vi "d7seg.vi"(0 "Numeric":u8 max=9 step=1) -> (19 "appended array":bool[](array[boolean]), 20 "a":bool, 21 "b":bool, 22 "c":bool, 23 "d":bool, 24 "e":bool, 25 "f":bool, 26 "g":bool, 27 "h":bool)   [LabVIEW 2023]
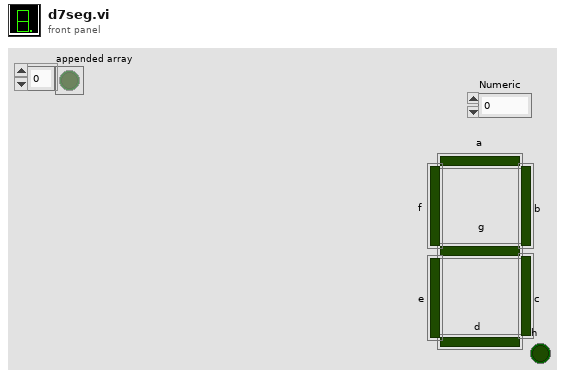
[diagram p1: front panel]
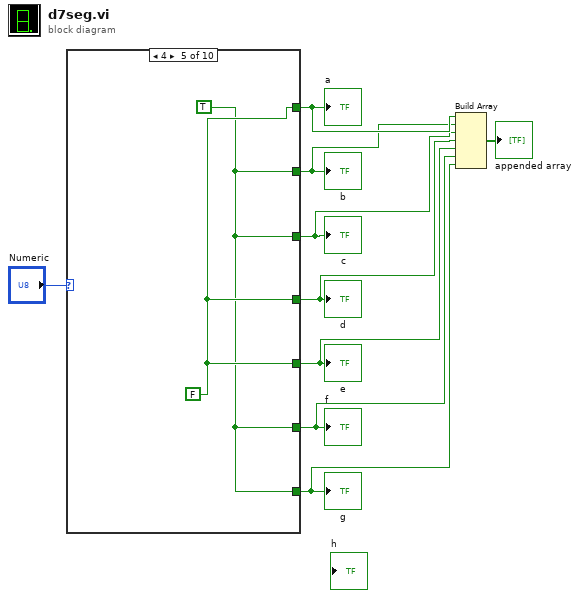
[diagram p0: block diagram]
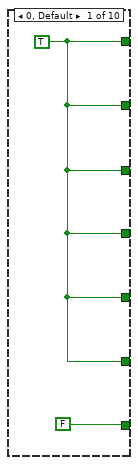
[diagram p2: hidden frame]
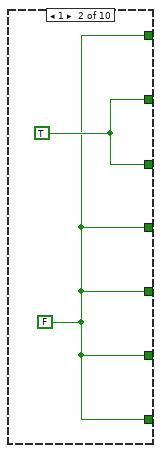
[diagram p3: hidden frame]
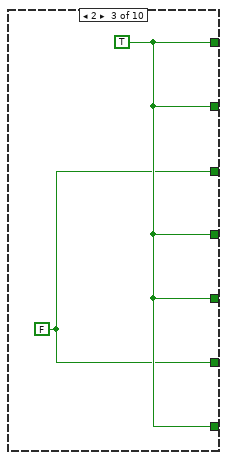
[diagram p4: hidden frame]
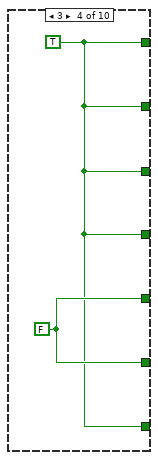
[diagram p5: hidden frame]
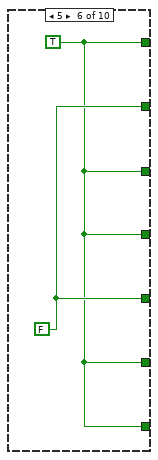
[diagram p6: hidden frame]
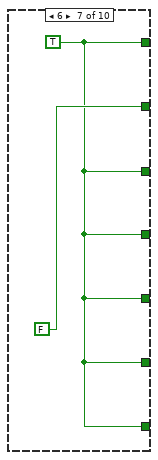
[diagram p7: hidden frame]
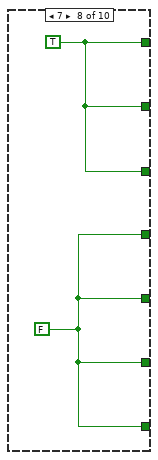
[diagram p8: hidden frame]
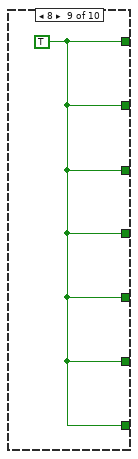
[diagram p9: hidden frame]
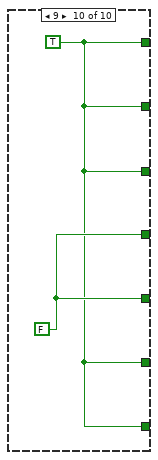
[diagram p10: hidden frame]
diagram:
  n1 = case shown="4" "Numeric" {
    tunnel: [w11 w12 w15 w16 w19 w20 w22 w25 w26 w27] -> w8
    tunnel: [w11 w13 w15 w16 w18 w21 FALSE w25 w26 w27] -> w7
    tunnel: [w11 w13 w14 w16 w18 w20 w22 w25 w26 w27] -> w6
    tunnel: [w11 w12 w15 w16 w19 w20 w22 w24 w26 w28] -> w5
    tunnel: [w11 w12 w15 w17 w19 w21 w22 w24 w26 w28] -> w4
    tunnel: [w11 w12 w14 w17 w18 w20 w22 w24 w26 w27] -> w3
    tunnel: [FALSE w12 w15 w16 w18 w20 w22 w24 w26 w27] -> w2
    frame 0, Default {
      w11 = TRUE
    }
    frame 1 {
      w12 = FALSE
      w13 = TRUE
    }
    frame 2 {
      w14 = FALSE
      w15 = TRUE
    }
    frame 3 {
      w17 = FALSE
      w16 = TRUE
    }
    frame 4 {
      w19 = FALSE
      w18 = TRUE
    }
    frame 5 {
      w21 = FALSE
      w20 = TRUE
    }
    frame 6 {
      w22 = TRUE
    }
    frame 7 {
      w24 = FALSE
      w25 = TRUE
    }
    frame 8 {
      w26 = TRUE
    }
    frame 9 {
      w28 = FALSE
      w27 = TRUE
    }
  }
  "a" <- w8
  "g" <- w2
  "d" <- w5
  "b" <- w7
  "c" <- w6
  "e" <- w4
  "f" <- w3
  n2 = Build Array(w8, w7, w6, w5, w4, w3, w2) -> (→"appended array":bool[])
